vi "test Read.vi"(11 "Test Case In":refnum<class "Test PCANBasic.lvclass">) -> (0 "error out":errorcluster, 3 "Test Case Out":refnum<class "Test PCANBasic.lvclass">)   [LabVIEW 2020, in "Test PCANBasic.lvclass"]
uses:
  Test PCANBasic.lvclass
  C:/Program Files/National Instruments/LabVIEW 2026/vi.lib/Astemes/LUnit/Test Case.lvclass
  <vilib>/Astemes/LUnit/Test Case.lvclass/Test Case.ctl
  source/PCANBasic.lvlib
  <vilib>/Astemes/LUnit/Test Case.lvclass
  Global PCAN Channel.vi
  Global PCAN Baudrate.vi
panel:
  out "Receive Queue empty":bool
  out "PCAN Message":T1 {"DATA"."7" format="%.0x"; "DATA"."6" format="%.0x"; "DATA"."5" format="%.0x"; "DATA"."4" format="%.0x"; "DATA"."3" format="%.0x"; "DATA"."2" format="%.0x"; "DATA"."1" format="%.0x"; "DATA"."0" format="%.0x"; "MSGTYPE"."Type" items=["STANDARD"=0, "RTR"=1, "ERRFRAME"=64, "STATUS"=128]}
  out "Time Stamp":timestamp format="%<%x %.3X>T"
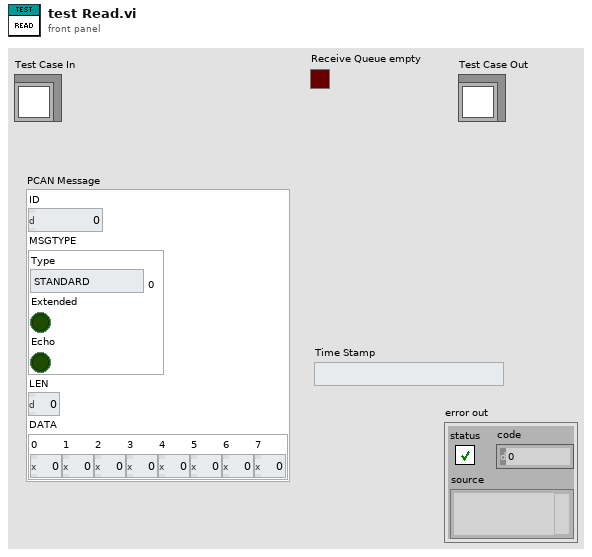
[diagram p1: front panel]
types:
  T1 = cluster{"ID":u32, "MSGTYPE":cluster{"Type":u8, "Extended":bool, "Echo":bool}, "LEN":u8, "DATA":cluster{"0":u8, "1":u8, "2":u8, "3":u8, "4":u8, "5":u8, "6":u8, "7":u8}}
  T2 = typedef "PCANBasic.lvlib/PCAN Baud.ctl" = u16
  T3 = typedef "PCANBasic.lvlib/TPCANHandle.ctl" = u16
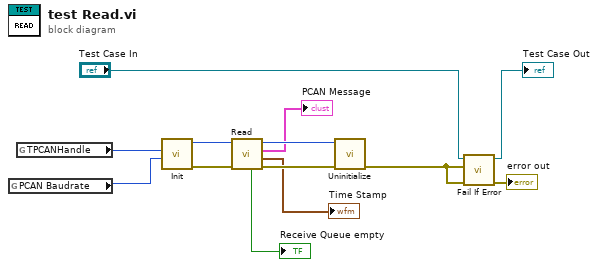
[diagram p0: block diagram]
diagram:
  n1 = global read "Global PCAN Baudrate.vi" "PCAN Baudrate"() -> (w3:T2)
  n2 = global read "Global PCAN Channel.vi" "TPCANHandle"() -> (w10:T3)
  n3 = call "Init.vi"("Baudrate"=w3, "Channel"=w10) -> ("error out"=w9:errorcluster, "TPCANHandle out"=w7:T3)  [unwired: 7 in, 1 out]
  n4 = call "Read.vi"("error in"=w9, "TPCANHandle in"=w7) -> ("error out"=w8:errorcluster, "Time Stamp"=→"Time Stamp":timestamp, "PCAN Message"=→"PCAN Message":T1, "TPCANHandle out"=w6:T3, "Receive Queue empty"=→"Receive Queue empty":bool)  [unwired: 4 in, 1 out]
  n5 = call "Uninitialize.vi"("error in"=w8, "TPCANHandle in"=w6) -> ("error out"=w4:errorcluster)  [unwired: 8 in, 1 out]
  n6 = call <vilib>:"Fail If Error.vi"("error in (no error)"=w4, "Assert error"=w4, "LUnit Test Case In"="Test Case In") -> ("error out"=→"error out":errorcluster, "LUnit Test Case Out"=→"Test Case Out":refnum<class "Test PCANBasic.lvclass">)  [unwired: 7 in]
